vi "Process-Postprocessing loop.vi"(8 "error":errorcluster, 9 "occurrence":refnum<k4>, 10 "Data-gen queue":T1, 11 "Queues Cluster":T2) -> ()   [LabVIEW 2017]
uses:
  User Interface/Queue/Message Queue/Typedefs/All Message Queues.ctl
  User Interface/Queue/Message Queue/Typedefs/Message Cluster.ctl
  Typedefs/Logging queue element.ctl
  Typedefs/Imaging Protocols enum.ctl
  Typedefs/Frame Size.ctl
  Typedefs/Acquired points count.ctl
  Logging/Typedefs/ROI File Generator Queue Ref.ctl
  Global Variables/General Globals.vi
panel:
  out "Abort":bool
  out "Last Trial Number":i32
  out "# elements in processing queue":i32
  out "ROI data loop rate (ms)":u32
  # "Background priority"
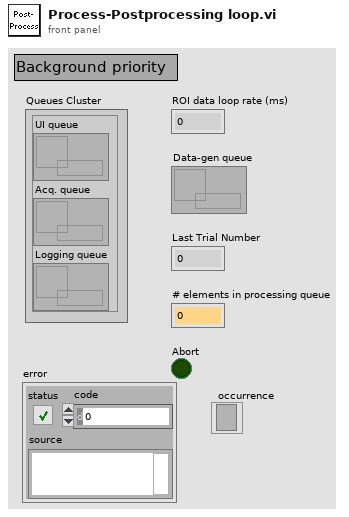
[diagram p1: front panel]
types:
  T1 = typedef "ROI File Generator Queue Ref.ctl" = refnum<queue>
  T2 = typedef "All Message Queues.ctl" = cluster{"UI queue":refnum<queue>, "Acq. queue":refnum<queue>, "Logging queue":refnum<queue>}
  T3 = typedef "Logging queue element.ctl" = cluster{"Imaging Protocol":T4, "Number of Trials":u16, "Frame Size":T5, "# Averaged frames":u16, "Dwell time (us)":dbl, "Index of Z-plane":i32, "Timelapse?":bool, "Logging process is active":bool, "Speed logging enabled":bool, "tdms file ref":refnum<k34>, "path":path, "Trial Number":i32, "Expected # points acquired":bool, "Manually stopped":bool, "Last trial":bool, "Ch0 data":u32[], "Ch1 data":u32[], "Ref Data":u32[], "Ref Frame Time":u64[], "Image Time":u64[], "Continuous Time":u64[], "Ref X Length":u16, "Ref Y Length":u16, "# Ref Averaged frames":u16, "Ref Dwell time (us)":dbl, "Points acquired":T6, "HW Timings File":refnum<file>}
  T4 = typedef "Imaging Protocols enum.ctl" = enum16{"AOL Z-Stack", "Motor Z Stack", "Functional Acquisition", "Single Plane Acquisition", "Volume Acquisition", "Live Imaging", "Live Plane Imaging", "Live Volume Imaging"}
  T5 = typedef "Frame Size.ctl" = u16
  T6 = typedef "Acquired points count.ctl" = cluster{"Ch0 last trial":u64, "Ch1 last trial":u64, "All trials":u64}
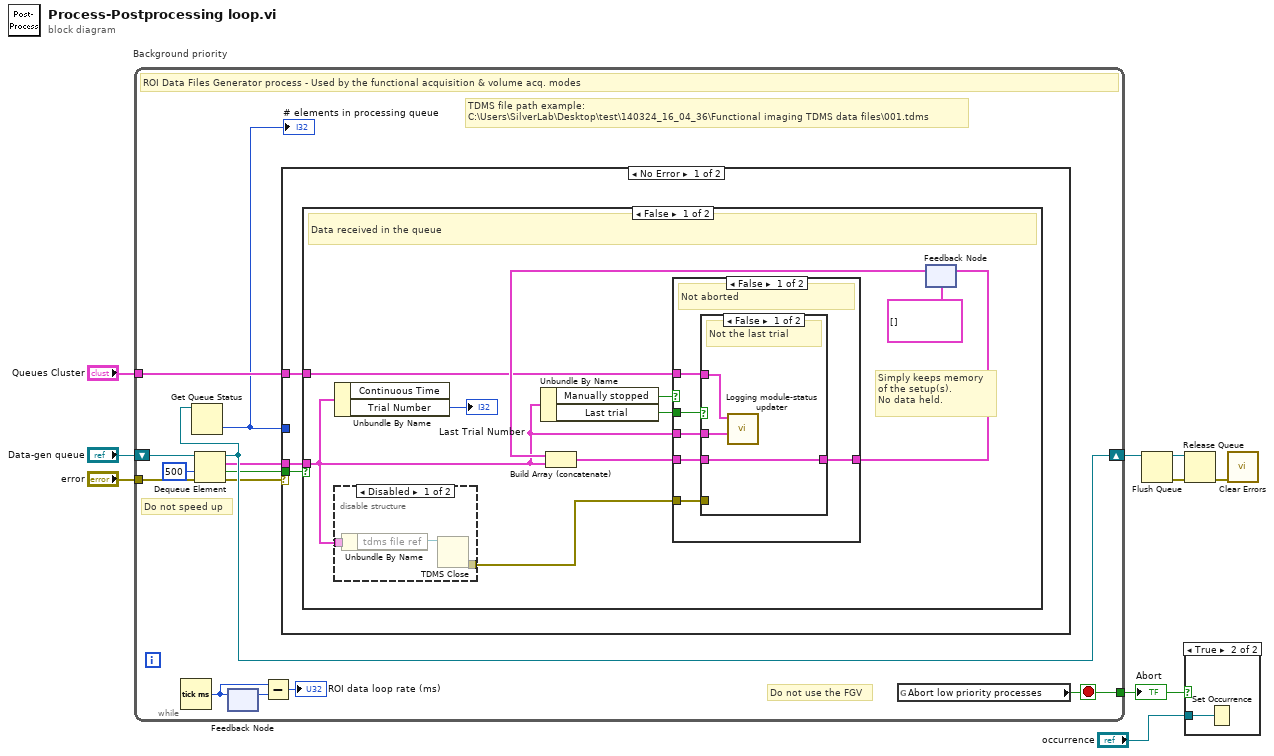
[diagram p0: block diagram]
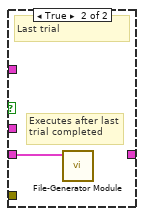
[diagram p3: hidden frame]
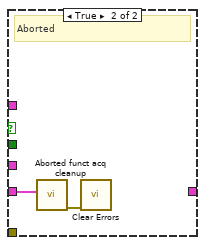
[diagram p4: hidden frame]
diagram:
  n1 = while "Background priority" {
    shift-right: [w19] -> w5
    shift-left: "Data-gen queue" -> [w22]
    tunnel: "error" -> [w21]
    tunnel: "Queues Cluster" -> [w20]
    tunnel: [w11] -> w2
    stop <- w11 stop-if-true
    # "Do not speed up"
    # "Do not use the FGV"
    # "TDMS file path example:\nC:\\Users\\SilverLab\\Desktop\\test\\140324_16_04_36\\Functional imaging TDMS data files\\001.tdms"
    # "ROI Data Files Generator process - Used by the functional acquisition & volume acq. modes"
    n2 = Tick Count (ms)() -> (millisecond timer value=w17:u32)
    n3 = Dequeue Element(queue=w22, timeout in ms (-1)=500, error in (no error)=w21) -> (queue out=w19:T1, element=w10:T3, timed out?=w14:bool, error out=w13:errorcluster)
    n4 = Get Queue Status(queue=w19) -> (# elements in queue=w12:i32)  [unwired: 2 in, 7 out]
    "# elements in processing queue" <- w12
    n5 = feedback #1() -> (w18:u32)  [unwired: 1 in]
    n6 = feedback-in #1(w17) -> ()
    n7 = Subtract(x=w17, y=w18) -> (x-y=→"ROI data loop rate (ms)":u32)
    n8 = case shown="No Error" w13 {
      tunnel: w10 -> [w23 _]
      tunnel: w14 -> [w25 _]
      tunnel: w12 -> [_ _]
      tunnel: w20 -> [w24 _]
      frame No Error {
        n9 = case shown="False" w25 {
          tunnel: w23 -> [w26 _]
          tunnel: w24 -> [w30 _]
          frame False {
            # "Simply keeps memory\nof the setup(s).\nNo data held."
            # "Data received in the queue"
            n10 = Unbundle By Name(w26) -> ("Trial Number"=→"Last Trial Number":i32)  [unwired: 1 out]
            n11 = disable-structure shown="Disabled" {
              disable-tunnel: w26 -> [w49 _]
              disable-tunnel: [w48 _] -> w29
              frame Disabled {
                n12 = Unbundle By Name(w49) -> ("tdms file ref"=w50:refnum<k34>)
                n13 = TDMS Close(11:w50) -> (0:w48:errorcluster)  [unwired: 1 in, 1 out]
              }
              frame Enabled {
                # "Closing a TDMS file takes a few seconds and hogs the CPU. So I moved the close function inside the file-gen module."
              }
            }
            n14 = Unbundle By Name(w26) -> ("Manually stopped"=w27:bool, "Last trial"=w35:bool)
            n15 = feedback #2(T3[] []) -> (w31:T3[])
            n16 = Build Array (concatenate)(w31, w26) -> (w32:T3[])
            n17 = case shown="False" w27 {
              tunnel: w35 -> [w41 _]
              tunnel: [w40 _] -> w34
              tunnel: w32 -> [w39 w46]
              tunnel: w30 -> [w38 _]
              tunnel: w29 -> [w37 _]
              tunnel: w26 -> [w36 _]
              frame False {
                # "Not aborted"
                n18 = case shown="False" w41 {
                  tunnel: [w44 _] -> w40
                  tunnel: w39 -> [w44 w45]
                  tunnel: w38 -> [w43 _]
                  tunnel: w36 -> [w42 _]
                  tunnel: w37 -> [_ _]
                  frame False {
                    # "Not the last trial"
                    n19 = call "Logging module-status updater.vi"("Queue element"=w42, "Message Queues"=w43) -> ()  [unwired: 9 in, 1 out]
                  }
                  frame True {
                    # "Executes after last\ntrial completed"
                    # "Last trial"
                    n20 = call "File-Generator Module.vi"("Metadata for all trials/volumes"=w45) -> ()  [unwired: 11 in]
                  }
                }
              }
              frame True {
                # "Aborted"
                n21 = call "Aborted funct acq cleanup.vi"("Metadata for all trials/volumes"=w46) -> ("error out"=w47:errorcluster)  [unwired: 10 in]
                n22 = call <vilib>:"Clear Errors.vi"("error in (no error)"=w47) -> ()  [unwired: 5 in, 2 out]
              }
            }
            n23 = feedback-in #2(w34) -> ()
          }
          frame True {
            # "Timed out (500ms). This case allows stopping the loop correctly."
          }
        }
      }
      frame Error {
      }
    }
    n24 = global read "General Globals.vi" "Abort low priority processes"() -> (w11:bool)
  }
  "Abort" <- w2
  n25 = Flush Queue(queue=w5) -> (queue out=w7:T1, error out=w6:errorcluster)  [unwired: 1 in, 1 out]
  n26 = Release Queue(queue=w7, error in (no error)=w6) -> (error out=w8:errorcluster)  [unwired: 1 in, 2 out]
  n27 = case shown="True" w2 {
    tunnel: "occurrence" -> [_ w51]
    frame False {
    }
    frame True {
      n28 = Set Occurrence(w51) -> ()
    }
  }
  n29 = call <vilib>:"Clear Errors.vi"("error in (no error)"=w8) -> ()  [unwired: 5 in, 2 out]
